vi "Sonicator Module (Main).vi"(7 "Name of Parent Panel":string="Main.vi", 9 "New Center Coords":T1={"Horizontal"=470, "Vertical"=200}, 10 "Config":variant, 11 "Main UI Message Queue":refnum<queue>) -> ()   [LabVIEW 2018, in "Sonicator Module.lvlib"]
doc: "This Continuous Measurement sample project is based on the Queued Message Handler template.\n\nThe Event Handling Loop generates messages based on user interface actions.\n\nThe Message Handling Loop processes messages generated by the Event Handling Loop, or by other messages. There are also Acquisition and Logging message handling loop subVIs, and a chart updating loop."
uses:
  Sonicator Module.lvlib
  support/Message Queue/Message Cluster.ctl
  <vilib>/Utility/miscctls.llb/LVPoint32TypeDef.ctl
  controls/UI State.ctl
  Feed Module/Controls/Sonicator Module Config Cluster.ctl
  Feed Module/Controls/Sonicator Module Settings Cluster.ctl
  Mettler Toledo/Controls/Settings Cluster.ctl
  Feed Module/Controls/Sonicator Module State Cluster.ctl
  Feed Module/Controls/Sonicator Module Display.ctl
  support/Message Queue/Enqueue Message (Single).vi
  support/User Event - Stop/User Event - Stop.lvlib
  support/Message Queue/Message Queue.lvlib
  support/Support Library.lvlib
  Measure Instrument/Sonicator Module Engine.lvlib
  Mettler Toledo/Mettler Toledo.lvlib
  Sonicator Settings Dialog.vi
  support/Command Log VIs/Command Logging.lvlib
panel:
  out "Ring":u16(ring)=2
  in  "Settings Button":bool
  out "ScanCode":i16
  out "µm":dbl format="%#_5f"
  out "Log File path":path
  out "Status":string
  in  "Exit":bool
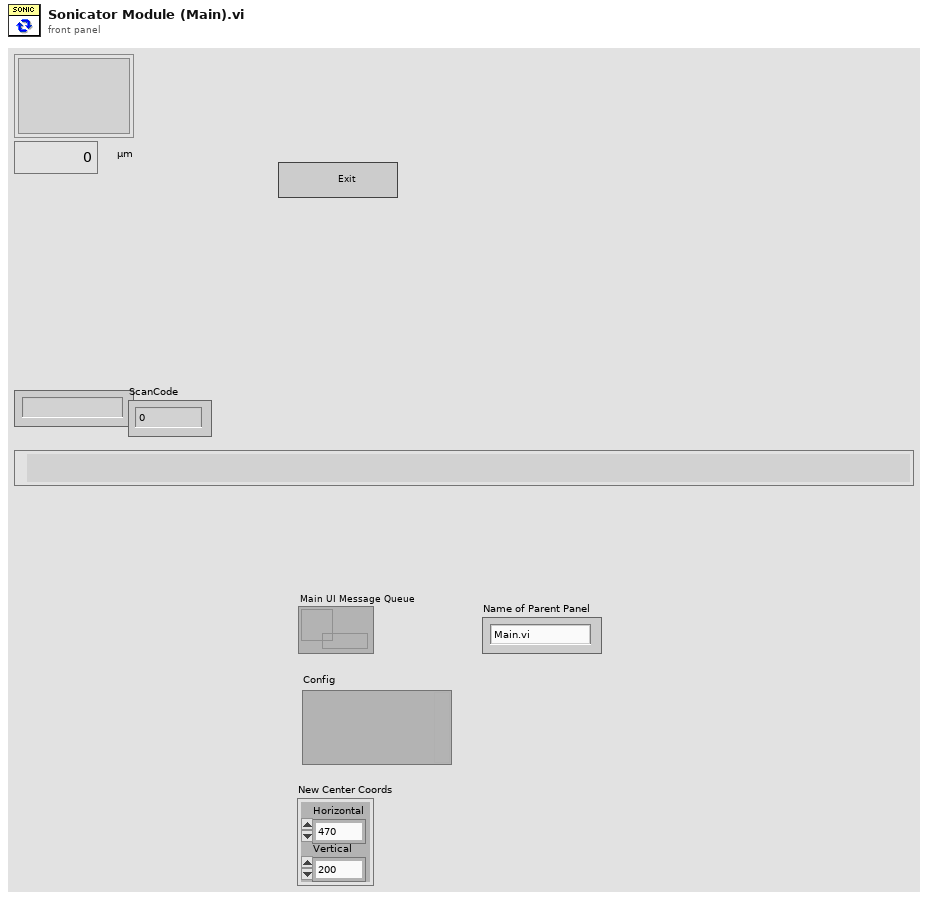
[diagram p1: front panel]
types:
  T1 = typedef "LVPoint32TypeDef.ctl" = cluster{"Horizontal":i32, "Vertical":i32}
  T2 = typedef "Sonicator Module.lvlib/Sonicator Module State Cluster.ctl" = cluster{"Scale Module Config":T3}
  T3 = typedef "Sonicator Module.lvlib/Sonicator Module Config Cluster.ctl" = cluster{"GUID":string, "Drop Coords":T1, "Process Name":string, "Queue Name":string, "Settings":T4, "Load Count":i32}
  T4 = typedef "Sonicator Module.lvlib/Sonicator Module Settings Cluster.ctl" = cluster{"Cycle Period":dbl, "Mettler":T5, "Scale Type":string}
  T5 = typedef "Mettler Toledo.lvlib/Settings Cluster.ctl" = cluster{"VISA resource name":refnum<visa-resource-name>, "Simulated?":bool}
  T6 = typedef "UI State.ctl" = enum16{"Idle", "Acquiring and Logging", "Waiting for Exit", "Waiting for Exit (Acq Stopped)", "Waiting for Exit (Log Stopped)", "Waiting for Stop", "Waiting for Stop (Acq Stopped)", "Waiting for Stop (Log Stopped)"}
  T7 = typedef "Sonicator Module.lvlib/Sonicator Message Queues.ctl" = cluster{"Sonicator UI":refnum<queue>, "Sonicator Engine":refnum<queue>, "Sonicator Display":refnum<queue>}
  T8 = typedef "Sonicator Module.lvlib/Sonicator Module Display.ctl" = cluster{"Pump On?":enum16{"Off", "On", "Not Initialized"}, "Sonicator Amp Value":dbl, "Sonicator Power Value":dbl, "Cycle Period":dbl}
  T9 = cluster{"Shift":bool, "Ctrl":bool, "Alt":bool, "Cmd":bool, "Opt":bool}
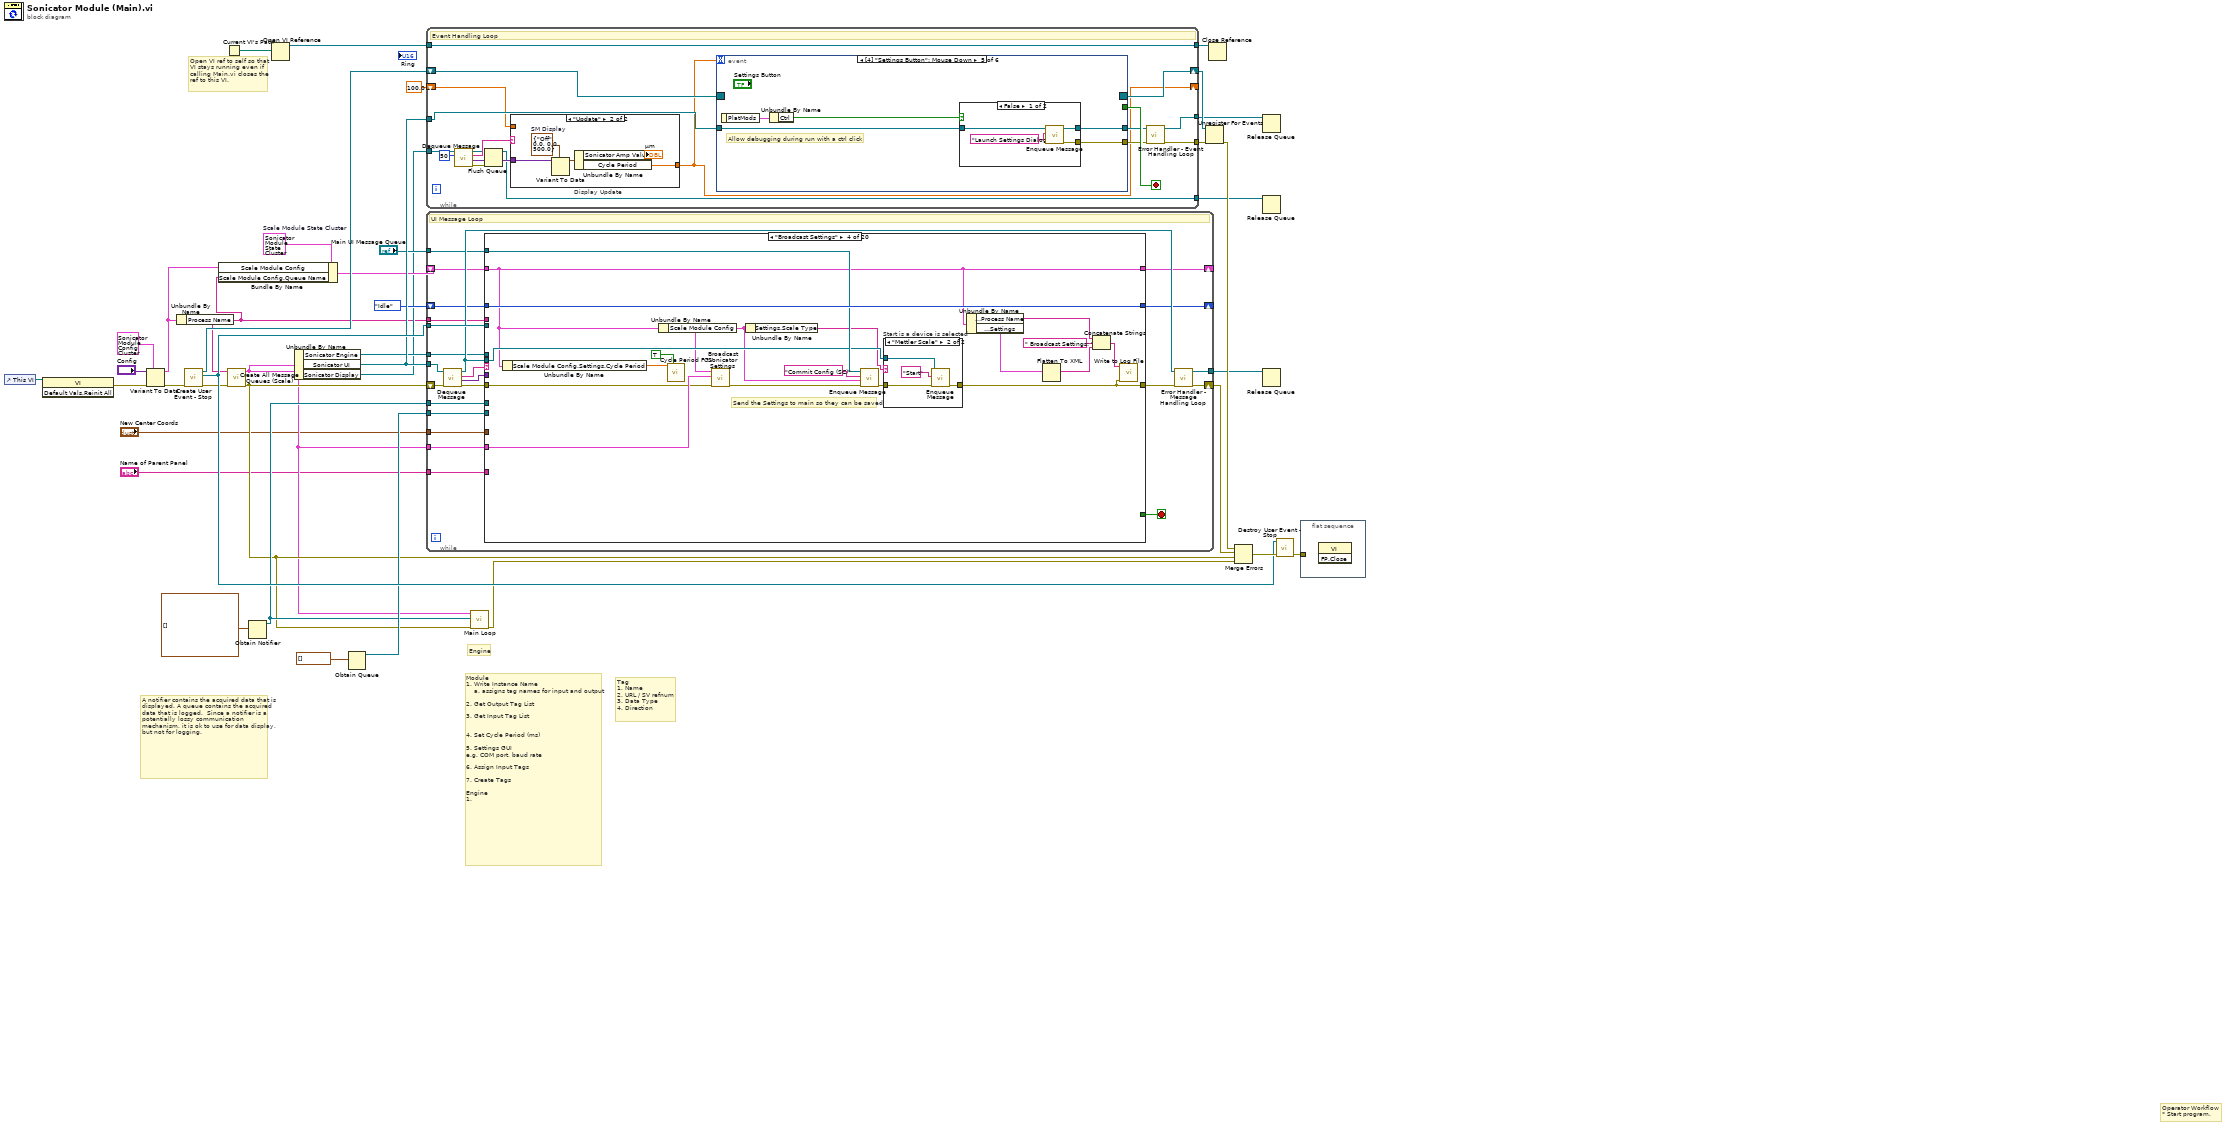
[diagram p0: block diagram]
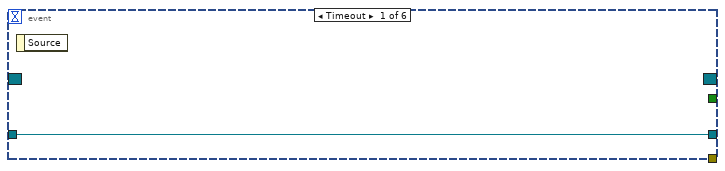
[diagram p3: hidden frame]
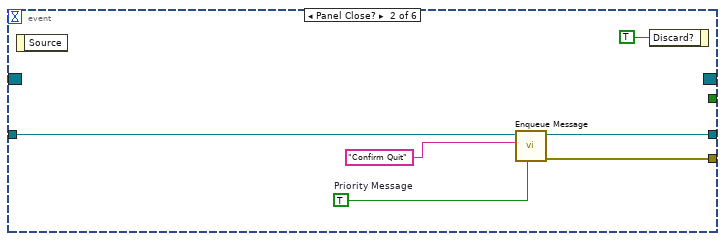
[diagram p4: hidden frame]
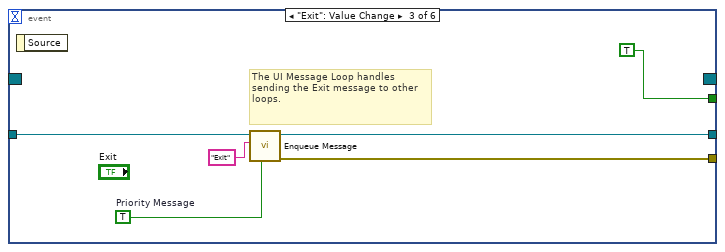
[diagram p5: hidden frame]
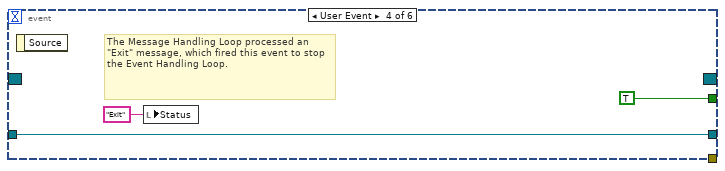
[diagram p6: hidden frame]
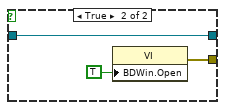
[diagram p7: hidden frame]
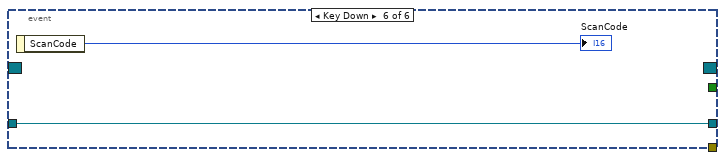
[diagram p8: hidden frame]
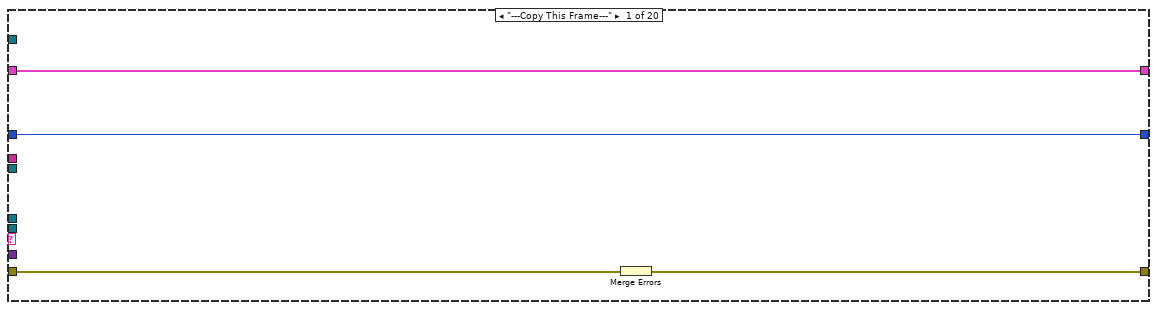
[diagram p9: hidden frame]
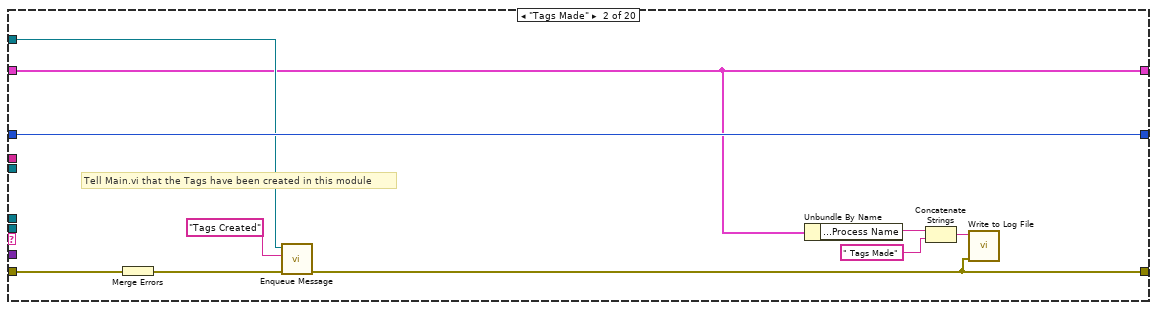
[diagram p10: hidden frame]
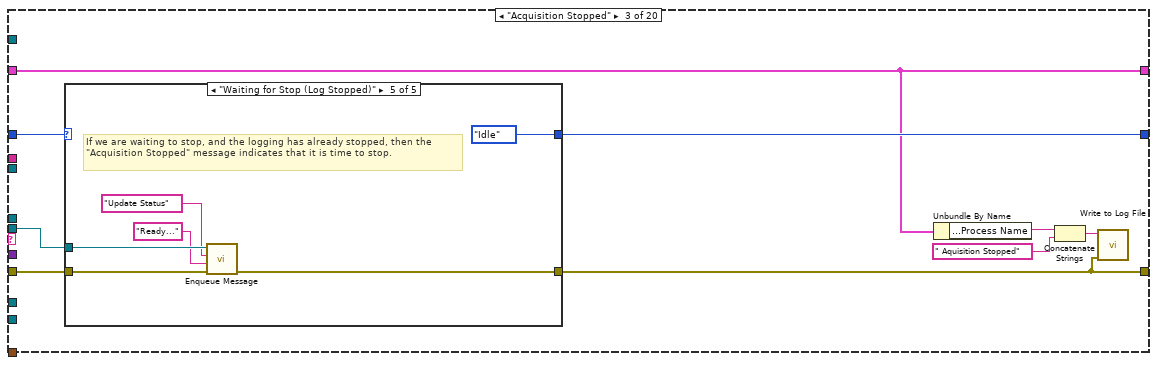
[diagram p11: hidden frame]
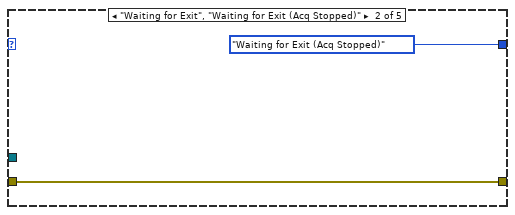
[diagram p13: hidden frame]
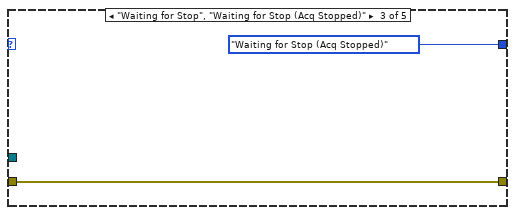
[diagram p14: hidden frame]
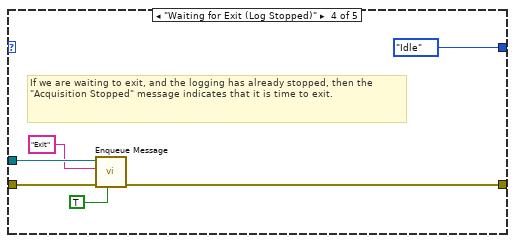
[diagram p15: hidden frame]
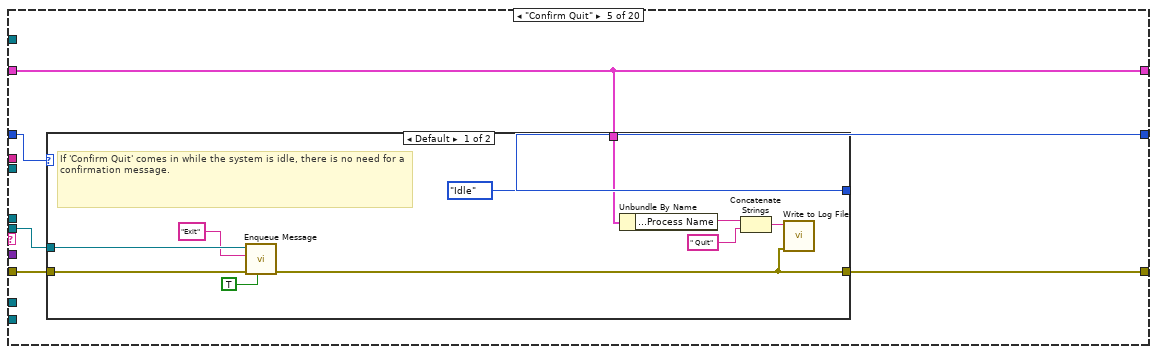
[diagram p17: hidden frame]
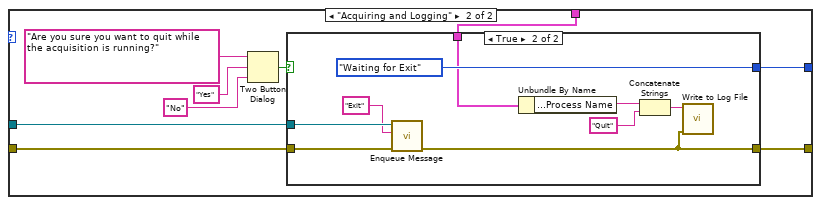
[diagram p18: hidden frame]
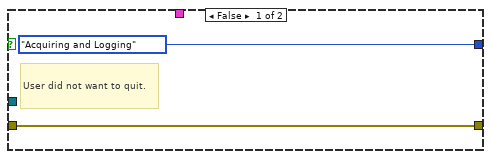
[diagram p19: hidden frame]
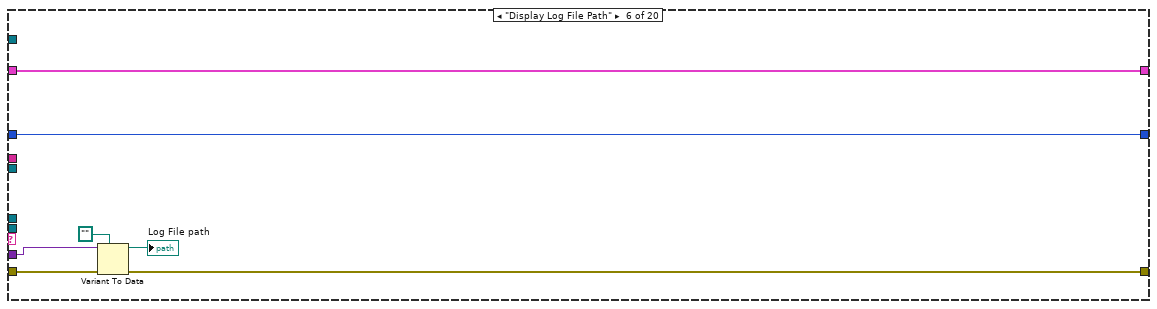
[diagram p20: hidden frame]
diagram:
  w17 = T2 {"Scale Module Config"={"GUID"="PID1-Mettler Toledo Scale 1", "Drop Coords"={"Horizontal"=0, "Vertical"=0}, "Process Name"="PID1-Setpoint", "Queue Name"="", "Settings"={"Cycle Period"=500.0, "Mettler"={"VISA resource name"="", "Simulated?"=FALSE}, "Scale Type"=""}, "Load Count"=0}}  # Scale Module State Cluster
  # "Open VI ref to self so that\nVI stays running even if\ncalling Main.vi closes the\nref to this VI."
  # "Engine"
  # "Operator Workflow\n* Start program."
  # "Module \n1. Write Instance Name\n    a. assigns tag names for input and output\n\n2. Get Output Tag List\n\n3. Get Input Tag List\n\n\n4. Set Cycle Period (ms)\n\n5. Settings GUI\ne.g. COM port, baud rate\n\n6. Assign Input Tags\n\n7. Create Tags\n\nEngine\n1."
  # "Tag\n1. Name\n2. URL / SV refnum\n3. Data Type\n4. Direction"
  # "A notifier contains the acquired data that is displayed. A queue contains the acquired data that is logged.  Since a notifier is a potentially lossy communication mechanism, it is ok to use for data display, but not for logging."
  n1 = control-ref of="This VI"() -> (w14:refnum<vi>)
  n2 = invoke class="VI" method="Default Vals.Reinit All"(reference=w14) -> (error out=w6:errorcluster)  [unwired: 2 in, 2 out]
  n3 = Variant To Data(error in=w6, type=T3 {"GUID"="", "Drop Coords"={"Horizontal"=0, "Vertical"=0}, "Process Name"="", "Queue Name"="", "Settings"={"Cycle Period"=500.0, "Mettler"={"VISA resource name"="", "Simulated?"=FALSE}, "Scale Type"=""}, "Load Count"=0} ("Feed Module Config"), Variant="Config") -> (data=w15:T3, error out=w20:errorcluster)
  n4 = Unbundle By Name(w15) -> ("Process Name"=w5:string)
  n5 = call "Create User Event - Stop.vi"("error in (no error)"=w20) -> ("error out"=w12:errorcluster, "User Event - Stop"=w35:refnum<user-event>, "Stop Event Registration Refnum"=w36:refnum<event-registration>)  [unwired: 8 in]
  n6 = Bundle By Name(cluster=w17, "Scale Module Config"=w15, "Scale Module Config.Queue Name"=w5) -> (w21:T2)
  n7 = Current VI's Path() -> (path=w22:path)
  n8 = call "Create All Message Queues (Scale).vi"("error in (no error)"=w12, "Process Name"=w5) -> ("error out"=w11:errorcluster, "Message Queues"=w10:T7)  [unwired: 8 in]
  n9 = Obtain Notifier(notification data type=waveform(dbl)[] []) -> (notifier out=w25:refnum<notifier>)  [unwired: 3 in, 2 out]
  n10 = Open VI Reference(vi path=w22) -> (vi reference=w23:refnum<vi>)  [unwired: 5 in, 1 out]
  n11 = Unbundle By Name(w10) -> ("Sonicator Engine"=w28:refnum<queue>, "Sonicator UI"=w32:refnum<queue>, "Sonicator Display"=w16:refnum<queue>)
  n12 = Obtain Queue(element data type=waveform(dbl)[] []) -> (queue out=w27:refnum<queue>)  [unwired: 4 in, 2 out]
  n13 = while {
    tunnel: w32 -> [w57]
    tunnel: w35 -> [w61]
    shift-right: [w53] -> w39
    shift-left: w11 -> [w60]
    shift-right: [w44] -> _
    shift-left: w21 -> [w46]
    tunnel: w25 -> [w56]
    tunnel: w27 -> [w55]
    shift-right: [w50] -> _
    shift-left: UI_State."Idle" ("UI State") -> [w51]
    tunnel: w28 -> [w49]
    tunnel: w10 -> [w48]
    tunnel: "Main UI Message Queue" -> [w45]
    tunnel: w5 -> [w43]
    tunnel: "New Center Coords" -> [w42]
    tunnel: "Name of Parent Panel" -> [w41]
    tunnel: [w40] -> w1
    stop <- w62 stop-if-true
    # "UI Message Loop"
    n14 = call "Dequeue Message.vi"("error in (no error)"=w60, "Message Queue"=w57) -> ("error out"=w47:errorcluster, "Message Data"=w58:variant, "Message"=w59:string, "dup Message Queue"=w52:refnum<queue>)  [unwired: 6 in]
    n15 = case "Message Cases" shown="\"Broadcast Settings\"" w59 {
      selector: w59 -> [_ _ _ _ _ _ _ _ _ _ _ _ _ _ _ _ _ _ _ w390]
      tunnel: w52 -> [_ _ w82 w114 w132 _ w182 w196 w218 _ w257 w273 w293 _ w331 _ _ w378 _ _]
      tunnel: w47 -> [w66 w76 w83 w118 w131 w166 w177 w200 w217 w243 w253 w272 w294 w317 w330 w335 w348 w373 w387 _]
      tunnel: [w65 w67 w78 w107 w130 w167 w172 w187 w202 w243 w245 w266 w289 w320 w326 w342 w350 w365 w388 w389] -> w54
      tunnel: [_ _ _ _ _ _ _ _ TRUE _ _ _ _ _ _ _ _ _ _ _] -> w62
      tunnel: w58 -> [_ _ _ _ _ w169 _ w199 w207 _ _ _ _ w318 _ _ _ _ w386 _]
      tunnel: w61 -> [_ _ _ _ _ _ _ _ w228 _ _ _ _ _ _ _ _ _ _ _]
      tunnel: w46 -> [w63 w68 w77 w106 w128 w164 w171 w186 w201 w240 w244 w265 w288 w324 w325 w336 w349 w364 w381 w395]
      tunnel: w56 -> [_ _ _ _ _ _ _ _ w226 _ _ _ _ _ _ _ _ _ _ _]
      tunnel: w55 -> [_ _ _ _ _ _ _ _ w222 _ _ _ _ _ _ _ _ _ _ _]
      tunnel: w51 -> [w64 w75 w85 w122 w133 w165 w178 w191 w215 _ _ w274 w296 w323 _ _ _ w374 w382 w399]
      tunnel: [w64 w75 w84 w122 w129 w165 w179 w191 w214 UI_State."Idle" ("UI State") UI_State."Idle" ("UI State") w274 w295 w323 UI_State."Acquiring and Logging" ("UI State") UI_State."Acquiring and Logging" ("UI State") UI_State."Acquiring and Logging" ("UI State") w375 w382 w399] -> w50
      tunnel: w49 -> [_ _ _ _ _ _ _ _ w221 _ _ _ _ _ _ w340 w357 w372 _ _]
      tunnel: w48 -> [_ _ _ w121 _ _ _ _ _ _ _ _ _ _ _ _ _ _ _ _]
      tunnel: w45 -> [_ w72 _ w115 _ _ _ _ w206 _ _ _ _ _ _ _ _ _ _ _]
      tunnel: [w63 w68 w77 w106 w128 w164 w171 w186 w201 w240 w244 w264 w288 w324 w325 w336 w349 w364 w381 w395] -> w44
      tunnel: w43 -> [_ _ _ _ _ _ _ _ _ _ w251 _ _ _ _ _ _ _ _ _]
      tunnel: w42 -> [_ _ _ _ _ _ _ _ _ _ w250 _ _ _ _ _ _ _ _ _]
      tunnel: w41 -> [_ _ _ _ _ _ _ _ _ _ w249 _ _ _ _ _ _ _ _ _]
      frame "---Copy This Frame---" {
        # "Duplicate this frame when creating new messages.  Change this comment in the duplicated frame to describe this message."
        n16 = Merge Errors(w66) -> (w65:errorcluster)
      }
      frame "Tags Made" {
        # "Tell Main.vi that the Tags have been created in this module"
        # "Duplicate this frame when creating new messages.  Change this comment in the duplicated frame to describe this message."
        n17 = Merge Errors(w76) -> (w73:errorcluster)
        n18 = call-poly "Enqueue Message.vi"("error in (no error)"=w73, "Message"="Tags Created", "Message Queue"=w72) -> ("error out"=w67:errorcluster)  [unwired: 7 in, 1 out]
        n19 = Unbundle By Name(w68) -> ("Scale Module Config.Process Name"=w71:string)
        n20 = Concatenate Strings(w71, " Tags Made" ("text")) -> (w69:string)
        n21 = call "Write to Log File.vi"("error in"=w67, "text"=w69) -> ()  [unwired: 9 in, 1 out]
      }
      frame "Acquisition Stopped" {
        # "Logic for determining what action to take when the acquisition has stopped."
        n22 = case shown="\"Waiting for Stop (Log Stopped)\"" w85 {
          selector: w85 -> [w87 _ _ _ _]
          tunnel: [w87 UI_State."Waiting for Exit (Acq Stopped)" ("UI State") UI_State."Waiting for Stop (Acq Stopped)" ("UI State") UI_State."Idle" ("UI State") UI_State."Idle" ("UI State")] -> w84
          tunnel: w83 -> [w86 w88 w90 w96 w102]
          tunnel: [w86 w88 w90 w95 w101] -> w78
          tunnel: w82 -> [_ _ _ w94 w100]
          frame Default {
          }
          frame "Waiting for Exit", "Waiting for Exit (Acq Stopped)" {
          }
          frame "Waiting for Stop", "Waiting for Stop (Acq Stopped)" {
          }
          frame "Waiting for Exit (Log Stopped)" {
            # "If we are waiting to exit, and the logging has already stopped, then the \"Acquisition Stopped\" message indicates that it is time to exit."
            n23 = call-poly "Enqueue Message.vi"("Priority Message? (F)"=TRUE, "error in (no error)"=w96, "Message"="Exit", "Message Queue"=w94) -> ("error out"=w95:errorcluster)  [unwired: 6 in, 1 out]
          }
          frame "Waiting for Stop (Log Stopped)" {
            # "If we are waiting to stop, and the logging has already stopped, then the \"Acquisition Stopped\" message indicates that it is time to stop."
            n24 = call-poly "Enqueue Message.vi"("error in (no error)"=w102, "Message Data"="Ready..." ("Message"), "Message"="Update Status", "Message Queue"=w100) -> ("error out"=w101:errorcluster)  [unwired: 6 in, 1 out]
          }
        }
        n25 = Unbundle By Name(w77) -> ("Scale Module Config.Process Name"=w81:string)
        n26 = Concatenate Strings(w81, " Aquisition Stopped" ("text")) -> (w79:string)
        n27 = call "Write to Log File.vi"("error in"=w78, "text"=w79) -> ()  [unwired: 9 in, 1 out]
      }
      frame "Broadcast Settings" {
        # "Send the Settings to main so they can be saved"
        # "Send the 'Update Settings' message to the Logging and Acquisition message loops."
        n28 = Unbundle By Name(w106) -> ("Scale Module Config.Settings.Cycle Period"=w119:dbl)
        n29 = Unbundle By Name(w106) -> ("Scale Module Config"=w111:T3)
        n30 = call "Cycle Period FGV.vi"("Write"=TRUE, "Cycle Period In (ms)"=w119) -> ()  [unwired: 8 in, 2 out]
        n31 = call "Broadcast Sonicator Settings.vi"("error in (no error)"=w118, "Message Queues"=w121, "Scale Module Config"=w111) -> ("error out"=w116:errorcluster)  [unwired: 8 in]
        n32 = Unbundle By Name(w111) -> ("Settings.Scale Type"=w112:string)
        n33 = call-poly "Enqueue Message.vi"("error in (no error)"=w116, "Message Data"=w111, "Message"="Commit Config (SC)", "Message Queue"=w115) -> ("error out"=w113:errorcluster)  [unwired: 6 in, 1 out]
        n34 = case "Start is a device is selected" shown="\"Mettler Scale\"" w112 {
          tunnel: w114 -> [_ w126]
          tunnel: w113 -> [w123 w125]
          tunnel: [w123 w124] -> w107
          frame "False", Default {
          }
          frame "Mettler Scale" {
            n35 = call-poly "Enqueue Message.vi"("error in (no error)"=w125, "Message"="Start", "Message Queue"=w126) -> ("error out"=w124:errorcluster)  [unwired: 7 in, 1 out]
          }
        }
        n36 = Unbundle By Name(w106) -> ("Scale Module Config.Process Name"=w110:string, "Scale Module Config.Settings"=w105:T4)
        n37 = Flatten To XML(anything=w105) -> (xml string=w104:string)
        n38 = Concatenate Strings(w110, " Broadcast Settings: " ("text"), w104) -> (w108:string)
        n39 = call "Write to Log File.vi"("error in"=w107, "text"=w108) -> ()  [unwired: 9 in, 1 out]
      }
      frame "Confirm Quit" {
        # "Confirm Quit - Message that can confirm whether or not the user wants to exit the application."
        n40 = case shown="Default" w133 {
          tunnel: w132 -> [w142 w149]
          tunnel: w131 -> [w141 w147]
          tunnel: [w135 w146] -> w130
          tunnel: [UI_State."Idle" ("UI State") w145] -> w129
          tunnel: w128 -> [w134 w144]
          frame Default {
            # "If 'Confirm Quit' comes in while the system is idle, there is no need for a confirmation message."
            n41 = call-poly "Enqueue Message.vi"("Priority Message? (F)"=TRUE, "error in (no error)"=w141, "Message"="Exit", "Message Queue"=w142) -> ("error out"=w135:errorcluster)  [unwired: 6 in, 1 out]
            n42 = Unbundle By Name(w134) -> ("Scale Module Config.Process Name"=w138:string)
            n43 = Concatenate Strings(w138, " Quit" ("text")) -> (w136:string)
            n44 = call "Write to Log File.vi"("error in"=w135, "text"=w136) -> ()  [unwired: 9 in, 1 out]
          }
          frame "Acquiring and Logging" {
            n45 = Two Button Dialog(message="Are you sure you want to quit while the acquisition is running?" ("Confirm Quit Message"), 1:"No" ("No"), 2:"Yes" ("Yes")) -> (T button?=w148:bool)
            n46 = case shown="True" w148 {
              tunnel: w149 -> [_ w163]
              tunnel: w147 -> [w153 w162]
              tunnel: [w153 w156] -> w146
              tunnel: [UI_State."Acquiring and Logging" ("UI State") UI_State."Waiting for Exit" ("UI State")] -> w145
              tunnel: w144 -> [_ w155]
              frame False {
                # "User did not want to quit."
              }
              frame True {
                n47 = call-poly "Enqueue Message.vi"("error in (no error)"=w162, "Message"="Exit", "Message Queue"=w163) -> ("error out"=w156:errorcluster)  [unwired: 7 in, 1 out]
                n48 = Unbundle By Name(w155) -> ("Scale Module Config.Process Name"=w159:string)
                n49 = Concatenate Strings(w159, "Quit" ("text")) -> (w157:string)
                n50 = call "Write to Log File.vi"("error in"=w156, "text"=w157) -> ()  [unwired: 9 in, 1 out]
              }
            }
          }
        }
      }
      frame "Display Log File Path" {
        n51 = Variant To Data(error in=w166, type=path "", Variant=w169) -> (data=→"Log File path":path, error out=w167:errorcluster)
      }
      frame "E-Stop" {
        # "E-Stop has no effect on the scale"
        # "Message Acquisition and Logging loops to stop"
        # "Stop the pumps."
        n52 = call-poly "Enqueue Message.vi"("error in (no error)"=w177, "Message Data"="Ready..." ("Ready..."), "Message"="Update Status", "Message Queue"=w182) -> ("error out"=w176:errorcluster)  [unwired: 6 in, 1 out]
        n53 = case shown="\"Waiting for Exit\"" w178 {
          selector: w178 -> [_ w184]
          tunnel: [UI_State."Waiting for Stop" ("UI State") w184] -> w179
          frame Default {
          }
          frame "Waiting for Exit" {
          }
        }
        n54 = Merge Errors(w176) -> (w172:errorcluster)
        n55 = Unbundle By Name(w171) -> ("Scale Module Config.Process Name"=w175:string)
        n56 = Concatenate Strings(w175, " E-STOP" ("text")) -> (w173:string)
        n57 = call "Write to Log File.vi"("error in"=w172, "text"=w173) -> ()  [unwired: 9 in, 1 out]
      }
      frame "Error" {
        # "Error - Check the error message data and respond accordingly. This message is sent by the \"Error Handler\" VIs at the end of each loop in this application."
        n58 = Variant To Data(error in=w200, type=errorcluster {"status"=FALSE, "code"=0, "source"=""} ("error out"), Variant=w199) -> (data=w197:errorcluster, error out=w193:errorcluster)
        n59 = call <vilib>:"General Error Handler.vi"("error in (no error)"=w197) -> ("message"=w185:string)  [unwired: 10 in, 4 out]
        n60 = call-poly "Enqueue Message.vi"("Priority Message? (F)"=TRUE, "Message"="Exit", "Message Queue"=w196) -> ("error out"=w192:errorcluster)  [unwired: 7 in, 1 out]
        n61 = Merge Errors(w192, w193) -> (w187:errorcluster)
        n62 = Unbundle By Name(w186) -> ("Scale Module Config.Process Name"=w190:string)
        n63 = Concatenate Strings(w190, " Error: " ("text"), w185) -> (w188:string)
        n64 = call "Write to Log File.vi"("error in"=w187, "text"=w188) -> ()  [unwired: 9 in, 1 out]
      }
      frame "Exit" {
        w210 = TRUE  # Delete Module?
        # "Don't check the error outs. The acquisition and logging queues may have already been released."
        # "Close references owned by the Main VI."
        # "Stop the VI"
        # "Exit - Fire the User Event to stop the Event Handling Loop.  Also send Exit messages to the Acquisition and Logging loops."
        n65 = call "Fire User Event - Stop.vi"("User Event - Stop"=w228) -> ("error out"=w227:errorcluster)  [unwired: 10 in]
        n66 = Build Array(w221) -> (w220:refnum<queue>[])
        n67 = for {
          tunnel: w220 -> [w237] mode=indexing
          n68 = call-poly "Enqueue Message.vi"("Message"="Stop", "Message Queue"=w237) -> ("dup Message Queue"=w238:refnum<queue>)  [unwired: 8 in, 1 out]
          n69 = call-poly "Enqueue Message.vi"("Message"="Exit", "Message Queue"=w238) -> ()  [unwired: 8 in, 2 out]
        }
        n70 = Variant To Data(type=w210, Variant=w207) -> (data=w209:bool, error out=w211:errorcluster)  [unwired: 1 in]
        n71 = call-poly "Enqueue Message.vi"("error in (no error)"=w217, "Message Data"="Ready..." ("Ready..."), "Message"="Update Status", "Message Queue"=w218) -> ("error out"=w216:errorcluster, "dup Message Queue"=w213:refnum<queue>)  [unwired: 6 in]
        n72 = Select(t=w210, s=w211, f=w209) -> (s? t:f=w208:bool)
        n73 = case "Don't enqueue Delete Module if opening campaign because it\nwill already have been deleted and new config loaded and we create\na race condition." shown="True" w208 {
          tunnel: w206 -> [_ w232]
          tunnel: w201 -> [_ w231]
          frame False {
          }
          frame True {
            n74 = Unbundle By Name(w231) -> ("Scale Module Config.GUID"=w230:string)
            n75 = call-poly "Enqueue Message.vi"("Message Data"=w230, "Message"="Delete Module", "Message Queue"=w232) -> ()  [unwired: 7 in, 2 out]
          }
        }
        n76 = Release Queue(queue=w213, error in (no error)=w216) -> (error out=w225:errorcluster)  [unwired: 1 in, 2 out]
        n77 = Release Notifier(notifier=w226, error in (no error)=w225) -> (error out=w224:errorcluster)  [unwired: 1 in, 2 out]
        n78 = Release Queue(queue=w222, error in (no error)=w224) -> (error out=w223:errorcluster)  [unwired: 1 in, 2 out]
        n79 = Merge Errors(w227, w223) -> (w202:errorcluster)
        n80 = case shown="Default" w215 {
          selector: w215 -> [_ w235]
          tunnel: [UI_State."Waiting for Stop" ("UI State") w235] -> w214
          frame Default {
          }
          frame "Waiting for Exit" {
          }
        }
        n81 = Unbundle By Name(w201) -> ("Scale Module Config.Process Name"=w205:string)
        n82 = Concatenate Strings(w205, " Exit" ("text")) -> (w203:string)
        n83 = call "Write to Log File.vi"("error in"=w202, "text"=w203) -> ()  [unwired: 9 in, 1 out]
      }
      frame "Init UI Refs" {
        # "Init UI Refs - Store control references for UI controls.  Also enable/disable controls appropriately."
        n84 = property class="VI"("Front Panel.Closeable"=TRUE ("Front Panel Window:Closeable")) -> ()  [unwired: 2 in, 2 out]
      }
      frame "Initialize" {
        # "Initialize - Get configuration settings, then message the UI to initialize, and broadcast the settings to the other message loops."
        n85 = call-poly "Enqueue Message.vi"("error in (no error)"=w253, "Message"="Init UI Refs", "Message Queue"=w257) -> ("error out"=w255:errorcluster, "dup Message Queue"=w256:refnum<queue>)  [unwired: 7 in]
        n86 = property class="VI" props=["FP.State"]() -> (reference out=w252:refnum<vi>)  [unwired: 2 in, 2 out]
        n87 = call "Make Child and Move.vi"("Process Name"=w251, "Name of Parent Panel"=w249, "New Center Coords"=w250, "VI in"=w252) -> ()  [unwired: 8 in]
        n88 = call-poly "Enqueue Message.vi"("error in (no error)"=w255, "Message"="Broadcast Settings", "Message Queue"=w256) -> ("error out"=w263:errorcluster, "dup Message Queue"=w262:refnum<queue>)  [unwired: 7 in]
        n89 = call-poly "Enqueue Message.vi"("error in (no error)"=w263, "Message Data"="Ready..." ("Ready..."), "Message"="Update Status", "Message Queue"=w262) -> ("error out"=w245:errorcluster)  [unwired: 6 in, 1 out]
        n90 = Unbundle By Name(w244) -> ("Scale Module Config.Process Name"=w248:string)
        n91 = Concatenate Strings(w248, " Initialize" ("text")) -> (w246:string)
        n92 = call "Write to Log File.vi"("error in"=w245, "text"=w246) -> ()  [unwired: 9 in, 1 out]
      }
      frame "Launch Settings Dialog" {
        # "Launch the Settings Dialog when the user clicks the 'Settings' button."
        n93 = in-place {
          in-place-border: w272 -> [w280]
          in-place-border: [w279] -> w271
          in-place-border: [w278] -> w270
          n94 = in-place-cluster #1(w265) -> ("Scale Module Config"=w276:T3)
          n95 = in-place {
            n96 = in-place-cluster #2(w276) -> ("Load Count"=w281:i32)
            n97 = Increment(x=w281) -> (x+1=w282:i32)
            n98 = in-place-cluster #2("Load Count"=w282) -> (w277:T3)
          }
          n99 = call-by-ref "?"("error in (no error)"=w280, "Scale Module Config In"=w277) -> ("error out"=w279:errorcluster, "Cancelled?"=w278:bool, "Scale Module Config Out"=w275:T3)  [unwired: 8 in, 3 out]
          n100 = in-place-cluster #1("Scale Module Config"=w275) -> (w264:T2)
        }
        n101 = case shown="False" w270 {
          tunnel: w271 -> [w284 w287]
          tunnel: [w283 w287] -> w266
          tunnel: w273 -> [w286 _]
          frame False {
            n102 = call-poly "Enqueue Message.vi"("error in (no error)"=w284, "Message"="Broadcast Settings", "Message Queue"=w286) -> ("error out"=w283:errorcluster)  [unwired: 7 in, 1 out]
          }
          frame True {
          }
        }
        n103 = Unbundle By Name(w264) -> ("Scale Module Config.Process Name"=w269:string)
        n104 = Concatenate Strings(w269, " Setting Dialog Launched" ("text")) -> (w267:string)
        n105 = call "Write to Log File.vi"("error in"=w266, "text"=w267) -> ()  [unwired: 9 in, 1 out]
      }
      frame "Logging Stopped" {
        # "Logic for determining what action to take when the logging has stopped."
        n106 = case shown="\"Waiting for Exit (Acq Stopped)\"" w296 {
          selector: w296 -> [w298 _ _ _ _]
          tunnel: [w298 UI_State."Waiting for Exit (Log Stopped)" ("UI State") UI_State."Waiting for Stop (Log Stopped)" ("UI State") UI_State."Idle" ("UI State") UI_State."Idle" ("UI State")] -> w295
          tunnel: w294 -> [w297 w299 w301 w307 w313]
          tunnel: [w297 w299 w301 w306 w312] -> w289
          tunnel: w293 -> [_ _ _ w305 w311]
          frame Default {
          }
          frame "Waiting for Exit", "Waiting for Exit (Log Stopped)" {
          }
          frame "Waiting for Stop", "Waiting for Stop (Log Stopped)" {
          }
          frame "Waiting for Exit (Acq Stopped)" {
            # "If we are waiting to exit, and the acquisition has already stopped, then the \"Logging Stopped\" message indicates that it is time to exit."
            n107 = call-poly "Enqueue Message.vi"("Priority Message? (F)"=TRUE, "error in (no error)"=w307, "Message"="Exit", "Message Queue"=w305) -> ("error out"=w306:errorcluster)  [unwired: 6 in, 1 out]
          }
          frame "Waiting for Stop (Acq Stopped)" {
            # "If we are waiting to stop, and the acquisition has already stopped, then the \"Logging Stopped\" message indicates that it is time to stop."
            n108 = call-poly "Enqueue Message.vi"("error in (no error)"=w313, "Message Data"="Ready..." ("Message"), "Message"="Update Status", "Message Queue"=w311) -> ("error out"=w312:errorcluster)  [unwired: 6 in, 1 out]
          }
        }
        n109 = Unbundle By Name(w288) -> ("Scale Module Config.Process Name"=w292:string)
        n110 = Concatenate Strings(w292, " Logging Stopped" ("text")) -> (w290:string)
        n111 = call "Write to Log File.vi"("error in"=w289, "text"=w290) -> ()  [unwired: 9 in, 1 out]
      }
      frame "Send to Sequence" {
        n112 = Variant To Data(error in=w317, type=refnum<queue> refnum ("Message Queue"), Variant=w318) -> (data=w315:refnum<queue>, error out=w316:errorcluster)
        n113 = local read "µm"() -> (w321:dbl)
        n114 = call-poly "Enqueue Message.vi"("error in (no error)"=w316, "Message Data"=w321, "Message"="Sent to Sequence", "Message Queue"=w315) -> ("error out"=w320:errorcluster)  [unwired: 6 in, 1 out]
      }
      frame "Start" {
        # "Message Acquisition and Logging loops to start"
        # "Start - Enable/Disable buttons appropriately for an acquisition that has started, and update status display."
        n115 = call-poly "Enqueue Message.vi"("error in (no error)"=w330, "Message"="Start Loops", "Message Queue"=w331) -> ("error out"=w332:errorcluster)  [unwired: 7 in, 1 out]
        n116 = Merge Errors(w332) -> (w326:errorcluster)
        n117 = Unbundle By Name(w325) -> ("Scale Module Config.Process Name"=w329:string)
        n118 = Concatenate Strings(w329, " Start" ("text")) -> (w327:string)
        n119 = call "Write to Log File.vi"("error in"=w326, "text"=w327) -> ()  [unwired: 9 in, 1 out]
      }
      frame "Start Loops" {
        # "I'm not sure what we would have multiple Process names in a module for but i'll leave it for now."
        # "Message Acquisition and Logging loops to start"
        # "Start - Enable/Disable buttons appropriately for an acquisition that has started, and update status display."
        n120 = Unbundle By Name(w336) -> ("Scale Module Config.Process Name"=w337:string)
        n121 = Build Array(w340) -> (w338:refnum<queue>[])
        n122 = property class="VI"("Front Panel.Title"=w337) -> ()  [unwired: 2 in, 2 out]
        n123 = for {
          tunnel: w335 -> [w346]
          tunnel: [w345] -> w339 mode=indexing
          tunnel: w338 -> [w344] mode=indexing
          tunnel: w337 -> [w343]
          n124 = call-poly "Enqueue Message.vi"("error in (no error)"=w346, "Message Data"=w343, "Message"="Start", "Message Queue"=w344) -> ("error out"=w345:errorcluster)  [unwired: 6 in, 1 out]
        }
        n125 = Merge Errors(w335, w339) -> (w342:errorcluster)
      }
      frame "Start Log" {
        # "I'm not sure what we would have multiple Process names in a module for but i'll leave it for now."
        # "Message Acquisition and Logging loops to start"
        # "Start - Enable/Disable buttons appropriately for an acquisition that has started, and update status display."
        n126 = Unbundle By Name(w349) -> ("Scale Module Config.Process Name"=w354:string)
        n127 = Build Array(w357) -> (w355:refnum<queue>[])
        n128 = property class="VI"("Front Panel.Title"=w354) -> ()  [unwired: 2 in, 2 out]
        n129 = for {
          tunnel: w348 -> [w362]
          tunnel: [w361] -> w356 mode=indexing
          tunnel: w355 -> [w360] mode=indexing
          tunnel: w354 -> [w359]
          n130 = call-poly "Enqueue Message.vi"("error in (no error)"=w362, "Message Data"=w359, "Message"="Start Log", "Message Queue"=w360) -> ("error out"=w361:errorcluster)  [unwired: 6 in, 1 out]
        }
        n131 = Merge Errors(w348, w356) -> (w350:errorcluster)
        n132 = Unbundle By Name(w349) -> ("Scale Module Config.Process Name"=w353:string)
        n133 = Concatenate Strings(w353, " Start Log" ("text")) -> (w351:string)
        n134 = call "Write to Log File.vi"("error in"=w350, "text"=w351) -> ()  [unwired: 9 in, 1 out]
      }
      frame "Stop" {
        # "Stop - Enable/Disable buttons appropriately for an acquisition that has stopped, and update status display."
        n135 = call-poly "Enqueue Message.vi"("error in (no error)"=w373, "Message Data"="Ready..." ("Ready..."), "Message"="Update Status", "Message Queue"=w378) -> ("error out"=w371:errorcluster)  [unwired: 6 in, 1 out]
        n136 = call-poly "Enqueue Message.vi"("error in (no error)"=w371, "Message"="Stop", "Message Queue"=w372) -> ("error out"=w369:errorcluster)  [unwired: 7 in, 1 out]
        n137 = case shown="Default" w374 {
          selector: w374 -> [_ w380]
          tunnel: [UI_State."Waiting for Stop" ("UI State") w380] -> w375
          frame Default {
          }
          frame "Waiting for Exit" {
          }
        }
        n138 = Merge Errors(w369) -> (w365:errorcluster)
        n139 = Unbundle By Name(w364) -> ("Scale Module Config.Process Name"=w368:string)
        n140 = Concatenate Strings(w368, " Stop" ("text")) -> (w366:string)
        n141 = call "Write to Log File.vi"("error in"=w365, "text"=w366) -> ()  [unwired: 9 in, 1 out]
      }
      frame "Update Status" {
        # "Update Display - Convert the message data to a string to display in the Status indicator."
        n142 = Variant To Data(error in=w387, type="", Variant=w386) -> (data=→"Status":string, error out=w384:errorcluster)
        n143 = Merge Errors(w384) -> (w388:errorcluster)
      }
      frame Default {
        # "'Default' case only runs if there is a message that isn't defined in any of the other cases.  Output a programming error."
        n144 = Concatenate Strings("The invalid message string " ("string"), w390, " was received in Scale Module Main" ("string")) -> (w391:string)
        n145 = Bundle By Name(cluster=errorcluster {"status"=TRUE, "code"=1, "source"=""} ("error constant"), "source"=w391) -> (w389:errorcluster)
        n146 = Unbundle By Name(w395) -> ("Scale Module Config.Process Name"=w398:string)
        n147 = Concatenate Strings(w398, "Invalid Message Recieved" ("text"), w390) -> (w396:string)
        n148 = call "Write to Log File.vi"("error in"=w389, "text"=w396) -> ()  [unwired: 9 in, 1 out]
      }
    }
    n149 = call "Error Handler - Message Handling Loop.vi"("error in (no error)"=w54, "Message Queue"=w52) -> ("dup error in"=w53:errorcluster, "dup Message Queue"=w40:refnum<queue>)  [unwired: 8 in]
  }
  n150 = while {
    tunnel: w32 -> [w411]
    tunnel: [w413] -> w38
    shift-right: [w412] -> w33
    shift-left: w36 -> [w417]
    tunnel: [w410] -> w24
    tunnel: w23 -> [w410]
    tunnel: w16 -> [w409]
    shift-right: [w406] -> _
    shift-left: 100.0 ("Cycle Period") -> [w405]
    tunnel: [w401] -> w3
    tunnel: [w400] -> w2
    stop <- w416 stop-if-true
    # "Event Handling Loop"
    n151 = call "Dequeue Message.vi"("timeout in ms (-1)"=50, "Message Queue"=w409) -> ("error out"=w402:errorcluster, "Message Data"=w407:variant, "Message"=w408:string, "dup Message Queue"=w403:refnum<queue>)  [unwired: 6 in]
    n152 = Flush Queue(queue=w403, error in (no error)=w402) -> (queue out=w400:refnum<queue>)  [unwired: 2 out]
    n153 = case "Display Update" shown="\"Update\"" w408 {
      tunnel: w407 -> [_ w423]
      tunnel: [w418 w420] -> w406
      tunnel: w405 -> [w418 _]
      frame "False", Default {
      }
      frame "Update" {
        w419 = T8 {"Pump On?"=enum."Off", "Sonicator Amp Value"=0.0, "Sonicator Power Value"=0.0, "Cycle Period"=500.0}  # SM Display
        n154 = Variant To Data(type=w419, Variant=w423) -> (data=w422:T8)  [unwired: 1 in, 1 out]
        n155 = Unbundle By Name(w422) -> ("Sonicator Amp Value"=→"µm":dbl, "Cycle Period"=w420:dbl)
      }
    }
    n156 = event shown="[4] \"Settings Button\": Mouse Down" {
      selector: w417 -> [_ _ _ _ _ _]
      dyn-events: [_ _ _ _ _ _] -> w412
      timeout: w406 -> [_ _ _ _ _ _]
      tunnel: [_ _ TRUE ("Discard?") TRUE ("Discard?") _ _] -> w416
      tunnel: w411 -> [w424 w427 w431 w437 w442 w452]
      tunnel: [_ w425 w436 _ w444 _] -> w414
      tunnel: [w424 w426 w434 w437 w443 w452] -> w415
      event Timeout {
        n157 = event-data() -> ()  [unwired: 1 in, 1 out]
      }
      event Panel Close? {
        w428 = TRUE  # Priority Message
        n158 = event-data() -> ()  [unwired: 1 in, 1 out]
        n159 = call-poly "Enqueue Message.vi"("Priority Message? (F)"=w428, "Message"="Confirm Quit", "Message Queue"=w427) -> ("error out"=w425:errorcluster, "dup Message Queue"=w426:refnum<queue>)  [unwired: 7 in]
        n160 = event-data("Discard?"=TRUE) -> ()  [unwired: 1 in, 1 out]
      }
      event "Exit": Value Change {
        w432 = TRUE  # Priority Message
        # "The UI Message Loop handles sending the Exit message to other loops."
        n161 = event-data() -> ()  [unwired: 1 in, 1 out]
        n162 = call-poly "Enqueue Message.vi"("Priority Message? (F)"=w432, "Message"="Exit", "Message Queue"=w431) -> ("error out"=w436:errorcluster, "dup Message Queue"=w434:refnum<queue>)  [unwired: 7 in]
      }
      event User Event {
        # "The Message Handling Loop processed an \"Exit\" message, which fired this event to stop the Event Handling Loop."
        n163 = event-data() -> ()  [unwired: 1 in, 1 out]
        n164 = local write "Status"("Exit" ("Exit String")) -> ()
      }
      event "Settings Button": Mouse Down {
        # "Allow debugging during run with a ctrl click"
        n165 = event-data() -> ("PlatMods"=w441:T9)  [unwired: 1 in]
        n166 = Unbundle By Name(w441) -> ("Ctrl"=w440:bool)
        n167 = case shown="False" w440 {
          tunnel: [w448 w449] -> w444
          tunnel: [w447 w450] -> w443
          tunnel: w442 -> [w446 w450]
          frame False {
            n168 = call-poly "Enqueue Message.vi"("Message"="Launch Settings Dialog", "Message Queue"=w446) -> ("error out"=w448:errorcluster, "dup Message Queue"=w447:refnum<queue>)  [unwired: 8 in]
          }
          frame True {
            n169 = property class="VI"("BDWin.Open"=TRUE ("Block Diagram Window:Open")) -> (error out=w449:errorcluster)  [unwired: 2 in, 1 out]
          }
        }
      }
      event Key Down {
        n170 = event-data() -> ("ScanCode"=→"ScanCode":i16)  [unwired: 1 in]
      }
    }
    n171 = call "Error Handler - Event Handling Loop.vi"("error in (no error)"=w414, "Message Queue"=w415) -> ("dup error in"=w413:errorcluster, "dup Message Queue"=w401:refnum<queue>)  [unwired: 8 in]
  }
  n172 = call "Main Loop.vi"("error in (no error)"=w11, "Chart Notifier"=w25, "Message Queues"=w10) -> ("error out"=w26:errorcluster)  [unwired: 8 in]
  n173 = Unregister For Events(event registration refnum=w33, error in=w38) -> (error out=w34:errorcluster)
  n174 = Close Reference(reference=w24) -> ()  [unwired: 1 in, 1 out]
  n175 = Merge Errors(w34, w39, w11, w26) -> (w37:errorcluster)
  n176 = Release Queue(queue=w3) -> ()  [unwired: 2 in, 3 out]
  n177 = Release Queue(queue=w2) -> ()  [unwired: 2 in, 3 out]
  n178 = Release Queue(queue=w1) -> ()  [unwired: 2 in, 3 out]
  n179 = call "Destroy User Event - Stop.vi"("error in (no error)"=w37, "User Event - Stop"=w35) -> ("error out"=w7:errorcluster)  [unwired: 9 in]
  n180 = flat-sequence {
    tunnel: w7 -> [_]
    frame #0 {
      n181 = invoke class="VI" method="FP.Close"() -> ()  [unwired: 3 in, 3 out]
    }
  }
